vi "String to Path (Linux convert).vi"(5 "Windows path":string) -> (2 "Path":path)   [LabVIEW 2019, in "BlueTOMLSerializer.lvlib"]
uses:
  BlueTOMLSerializer.lvlib
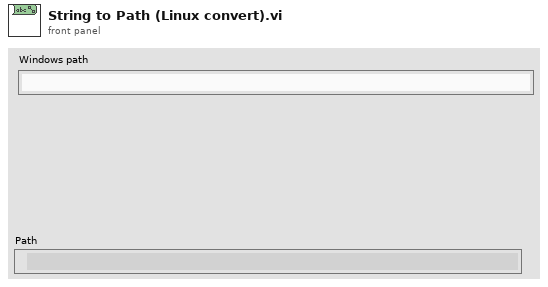
[diagram p1: front panel]
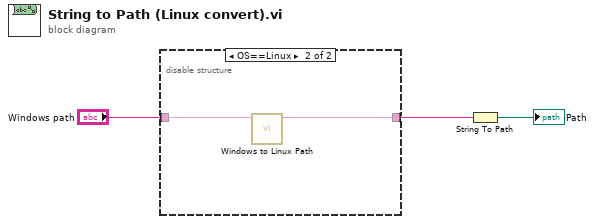
[diagram p0: block diagram]
diagram:
  n1 = disable-structure shown="OS==Linux" {
    disable-tunnel: "Windows path" -> [w4 w6]
    disable-tunnel: [w4 w5] -> w2
    frame condition #0 (active) {
    }
    frame condition #1 {
      n2 = call "Windows to Linux Path.vi"("Windows path"=w6) -> ("Linux Path"=w5:string)  [unwired: 9 in, 1 out]
    }
  }
  n3 = String To Path(string=w2) -> (path=→"Path":path)
